vi "Temperatura.vi"() -> ()   [LabVIEW 2025]
uses:
  <vilib>/Instr/_visa.llb/VISA Configure Serial Port (Instr).vi
panel:
  in  "Reset":bool
  in  "byte count":u32
  in  "VISA resource name":refnum<visa-resource-name>
  in  "stop":bool
  out "Waveform Chart":dbl(graph)
  out "Temperatura":dbl
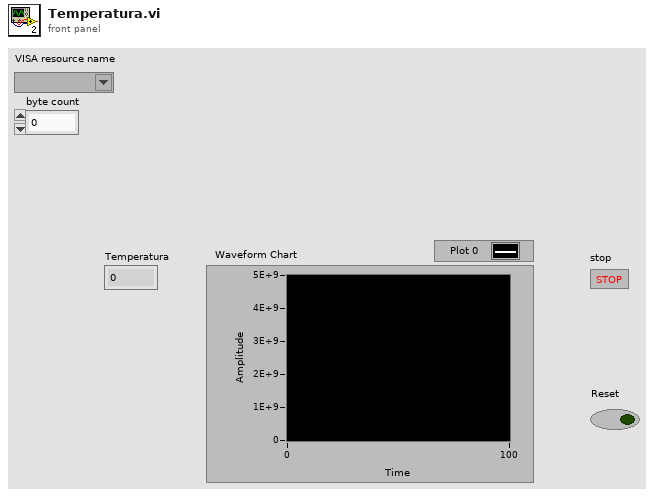
[diagram p1: front panel]
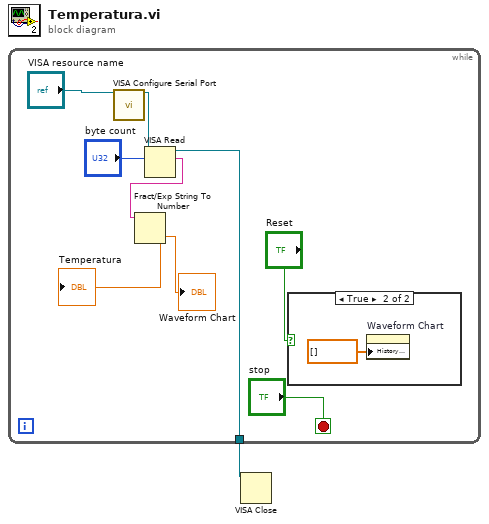
[diagram p0: block diagram]
diagram:
  n1 = while {
    tunnel: [w4] -> w1
    stop <- "stop" stop-if-true
    n2 = call-poly "VISA Configure Serial Port"("VISA resource name"="VISA resource name") -> ("VISA resource name out"=w8:refnum<visa-resource-name>)  [unwired: 13 in, 1 out]
    n3 = VISA Read(VISA resource name=w8, byte count="byte count") -> (VISA resource name out=w4:refnum<visa-resource-name>, read buffer=w6:string)  [unwired: 1 in, 2 out]
    n4 = Fract/Exp String To Number(string=w6) -> (number=→"Temperatura" →"Waveform Chart":dbl)  [unwired: 3 in, 1 out]
    n5 = case shown="True" "Reset" {
      frame False {
      }
      frame True {
        n6 = property on="Waveform Chart" class="WFChart (strict)"("History Data"=dbl[] []) -> ()  [unwired: 2 in, 2 out]
      }
    }
  }
  n7 = VISA Close(VISA resource name=w1) -> ()  [unwired: 1 in, 1 out]
